vi "Create Date Time String.vi"(8 "错误输入":cluster{"状态":bool, "代码":i32, "源":string}) -> (0 "错误输出":cluster{"状态":bool, "代码":i32, "源":string}, 2 "日期/时间字符串":string)   [LabVIEW 2012]
doc: "创建包含当前日期和时间的字符串（比如Apr-21-2012 Time 11 38 PM）。"
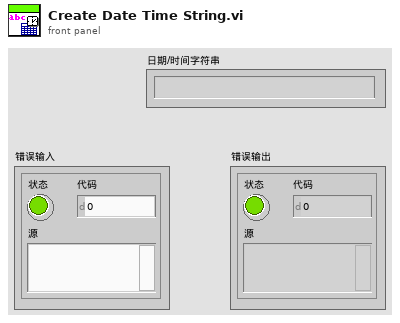
[diagram p1: front panel]
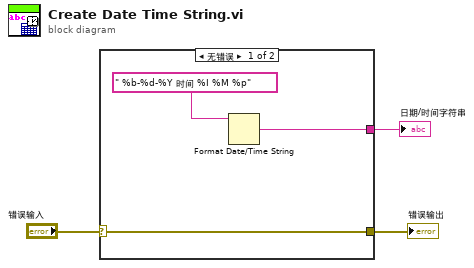
[diagram p0: block diagram]
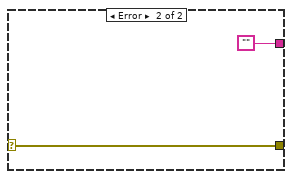
[diagram p2: hidden frame]
diagram:
  n1 = case shown="无错误" "错误输入" {
    selector: "错误输入" -> [w5 w7]
    tunnel: [w5 w7] -> w2
    tunnel: [w4 "" ("空字符串常量")] -> w1
    frame No Error {
      n2 = Format Date/Time String ("格式化日期/时间字符串")(time format string (%c)=" %b-%d-%Y 时间 %I %M %p" ("时间格式字符串(%c)")) -> (date/time string=w4:string)  [unwired: 2 in]
    }
    frame Error {
    }
  }
  "错误输出" <- w2
  "日期/时间字符串" <- w1
